vi "Periodic Tasks.vi"(8 "error in":errorcluster) -> (3 "Boolean":bool)   [LabVIEW 2023]
doc: "This VI runs in parallel to other tasks. It can contain as many user-defined periodic loops as you need. These can carry out PID or other sorts of timed response."
uses:
  Systems/SwerveDrive/SwerveDrive_ACT_ts.lvlib
  Systems/Game Controller/GameController_SEN.lvlib
  Systems/PigeonIMU/PigeonIMU_SEN_ts.lvlib
  Systems/Shooter/Shooter_ACT.lvlib
  Systems/2024 Intake/Intake_ACT.lvlib
  Systems/2024 ChainLift/ChainLift_ACT.lvlib
  Systems/2024 RingPlacer/RingPlacer_ACT.lvlib
  Systems/Elevator/2024 Elevator_ACT.lvlib
  Systems/Pivot FX/Pivot FX_ACT.lvlib
  Systems/AUTO 2023/2023-Auto_CMD.lvlib
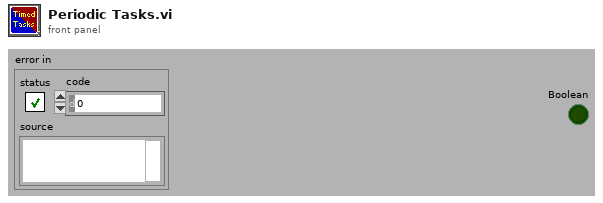
[diagram p1: front panel]
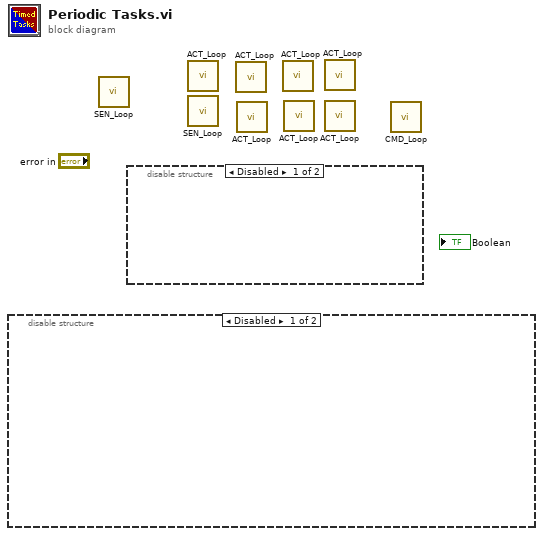
[diagram p0: block diagram]
diagram:
  n1 = disable-structure shown="Disabled" {
    frame Disabled {
    }
    frame Enabled {
    }
  }
  n2 = call "SEN_Loop.vi"() -> ()  [unwired: 12 in]
  n3 = disable-structure shown="Disabled" {
    frame Disabled {
    }
    frame Enabled {
    }
  }
  n4 = call "ACT_Loop.vi"() -> ()  [unwired: 12 in]
  n5 = call "SEN_Loop.vi"() -> ()  [unwired: 12 in]
  n6 = call "ACT_Loop.vi"() -> ()  [unwired: 12 in]
  n7 = call "ACT_Loop.vi"() -> ()  [unwired: 12 in]
  n8 = call "ACT_Loop.vi"() -> ()  [unwired: 12 in]
  n9 = call "ACT_Loop.vi"() -> ()  [unwired: 12 in]
  n10 = call "ACT_Loop.vi"() -> ()  [unwired: 12 in]
  n11 = call "ACT_Loop.vi"() -> ()  [unwired: 12 in]
  n12 = call "CMD_Loop.vi"() -> ()  [unwired: 12 in]
